vi "系统设置.vi"() -> ()   [LabVIEW 2016]
uses:
  <vilib>/Utility/miscctls.llb/LVPointTypeDef.ctl
  <vilib>/ptbypt/NI_PtbyPt.lvlib
  <vilib>/Utility/config.llb/NI_LVConfig.lvlib
  PLC/PLC.lvlib
  API/CodCr/CodCr.lvlib
panel:
  in  "超标留样启用":bool caption="质控单元禁用"
  in  "周期设置":enum16{"自由设定", "国标协议"}(ring)
  in  "运行间隔":i16=4 min=1 max=24
  out "x = y?":bool
  in  "质控启动日期":string(combo)="关闭"
  in  "跨度核查时间":u16(ring)=6 items=["00H", "01H", "02H", "03H", "04H", "05H", "06H", "07H", "08H", "09H", "10H", "11H", "12H", "13H", "14H", "15H", "16H", "17H", "18H", "19H", "20H", "21H", "22H", "23H"]
  in  "空白核查时间":u16(ring)=2 items=["00H", "01H", "02H", "03H", "04H", "05H", "06H", "07H", "08H", "09H", "10H", "11H", "12H", "13H", "14H", "15H", "16H", "17H", "18H", "19H", "20H", "21H", "22H", "23H"]
  in  "CODCr":bool
  in  "总磷总氮":bool
  in  "氨氮":bool
  in  "CODmn":bool
  in  "多参数":bool
  in  "24H周期设置":bool[](xcontrol)
  in  "输入密码":dbl
  in  "布尔":bool
  in  "副屏设置":bool
  in  "开机启动":bool caption="氨氮禁用"
  in  "CODMn启用":bool caption="CODMn禁用"
  in  "质控单元启用":bool caption="质控单元禁用"
  in  "总磷总氮启用":bool caption="总磷总氮禁用"
  in  "流量计启用":bool caption="流量计禁用"
  in  "氨氮启用":bool caption="氨氮禁用"
  in  "多参数启用":bool caption="多参数禁用"
  in  "CODcr启用":bool caption="CODcr禁用"
  in  "运行模式":enum16{"维护模式", "常规模式", "应急模式", "质控模式"}(ring)
  # "注：周期设置分为自由设定和国标协议两种。\n1：选择自由设定情况下：运行间隔将不可选用并变灰色，周期设置可自由手动勾选\n2：选择国标协议情况下：周期时间将由运行间隔选择的时间决定，下方周期设置被禁用并无法手动勾选。"
  # "自动运行启动参数"
  # "启动周期设置"
  # "质控频次："
  # "空白核查时间："
  # "跨度核查时间："
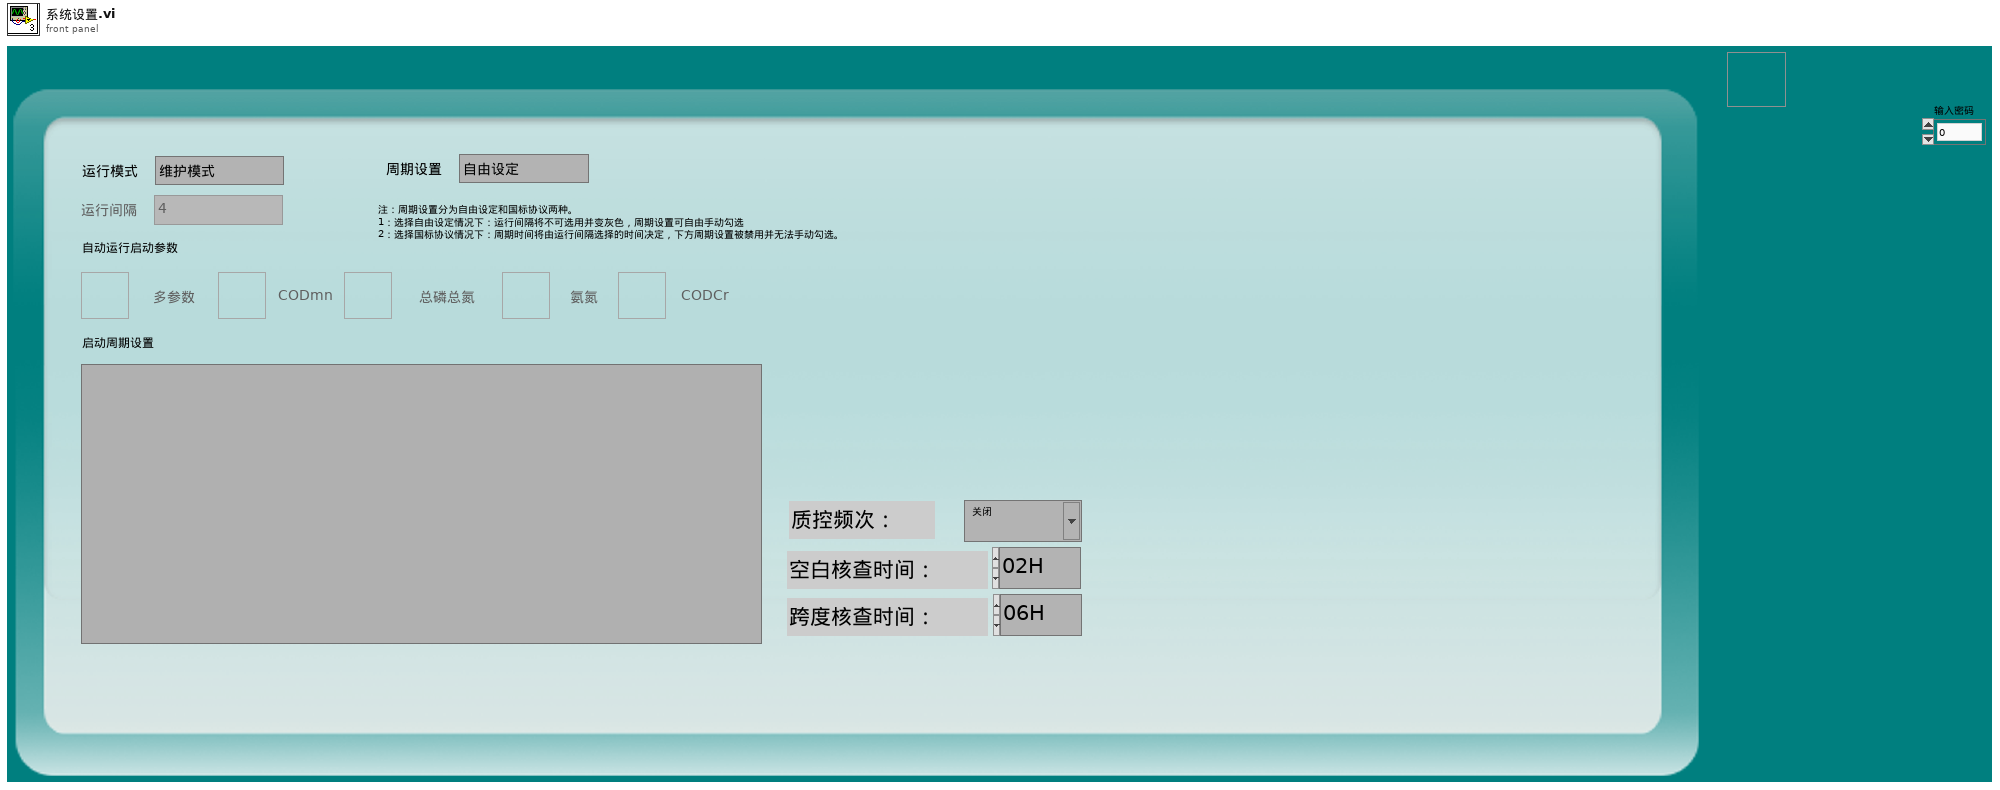
[diagram p1: front panel]
types:
  T1 = typedef "LVPointTypeDef.ctl" = cluster{"Horizontal":i16, "Vertical":i16}
  T2 = typedef "NI_LVConfig.lvlib/Config Data RefNum.ctl" = refnum<k1>
  T3 = enum8{"Enabled", "Disabled", "Disabled and Grayed Out"}
  T4 = enum32{"Invalid", "Standard", "Closed", "Hidden", "Minimized", "Maximized"}
  T5 = enum32{"Bad", "Idle", "Run top level", "Running"}
  T6 = cluster{"运行模式":enum16{"维护模式", "常规模式", "应急模式", "质控模式"}}
  T7 = cluster{"测量模式":enum16{"水样测量", "标样核查", "零点核查", "跨度核查", "加标回收", "平行样", "校零", "校标"}}
  T8 = cluster{"测量模式":enum16{"水样测量", "标样核查", "零点核查", "跨度核查", "空白测试", "加标回收", "平行样", "校零", "校标"}}
  T9 = cluster{"水样测试量程切换模式":enum16{"H", "L", "AUTO"}, "空白核查量程切换模式":enum16{"H", "L", "AUTO"}, "跨度核查量程切换模式":enum16{"H", "L", "AUTO"}}
  T10 = cluster{"站号":u16, "量程切换":enum32{"H", "L", "AUTO"}, "控制命令":enum16{"启动测量", "标样核查", "零点核查", "跨度核查", "空白测试", "平行样测试", "加标回收", "空白校准", "标样校准", "初始化（清洗）", "停止测试", "仪器重启", "校时", "模式设置", "测量间隔设置"}, "模式设置":enum16{"待机", "连续模式", "周期模式", "定点模式", "受控模式", "手动模式"}, "测量间隔":u16}
  T11 = cluster{"CODCr":cluster{"启动测量模式":cluster{"测量模式":enum16{"水样测量", "标样核查", "零点核查", "跨度核查", "加标回收", "平行样", "校零", "校标"}}, "确定按钮":bool}, "参数启用":cluster{"多参数":bool, "CODMn":bool, "总磷总氮":bool, "氨氮":bool, "CODcr":bool}}
  T12 = typedef "LVDateTimeRec.ctl" = cluster{"秒数的小数部分":dbl, "秒":i32, "分":i32, "时":i32, "日":i32, "月":i32, "年":i32, "天数（周）":i32, "天数（年）":i32, "DST":i32}
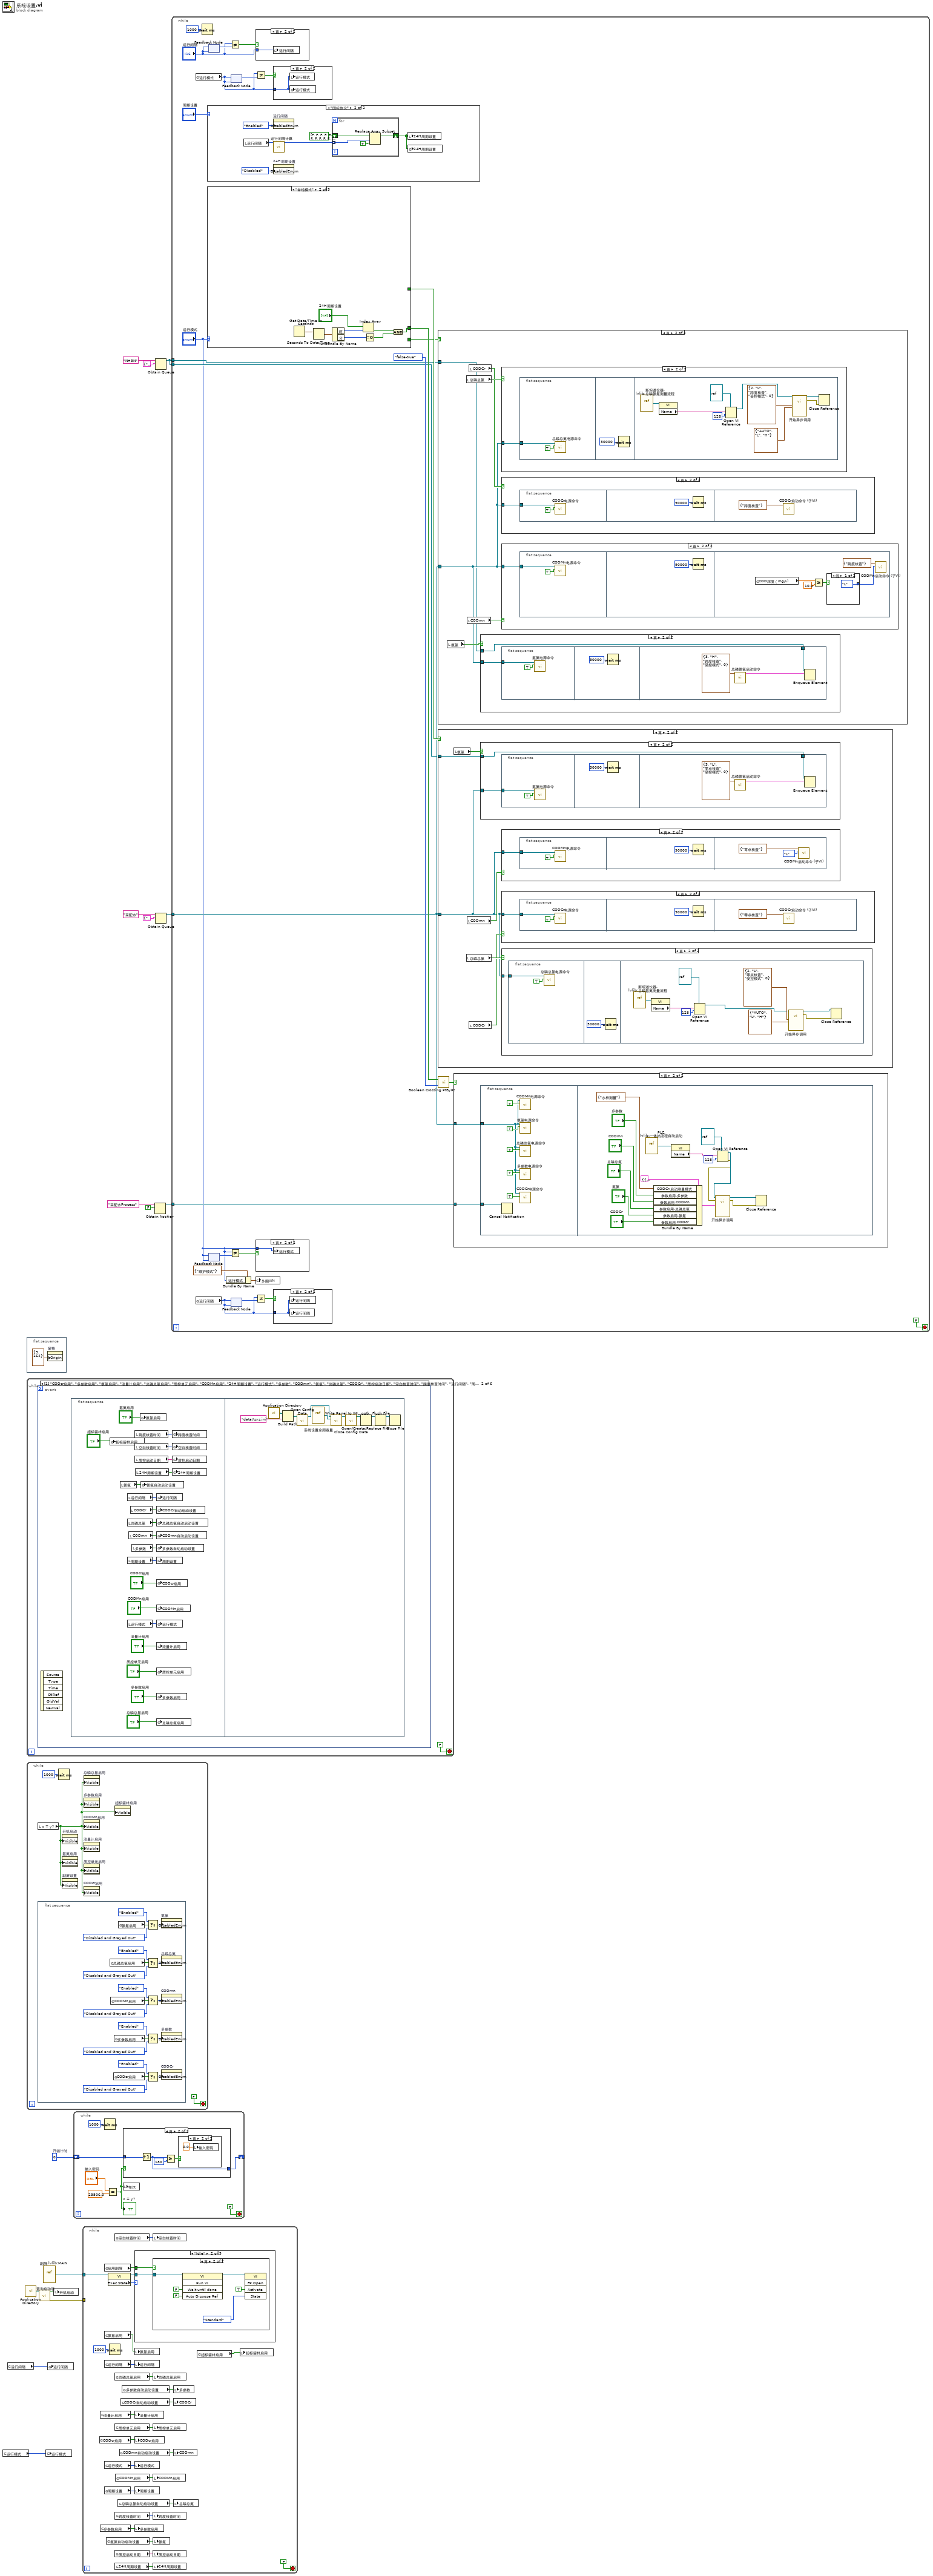
[diagram p0: block diagram]
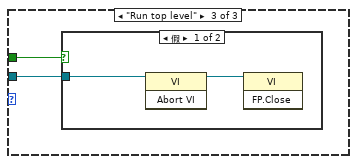
[diagram p6: hidden frame]
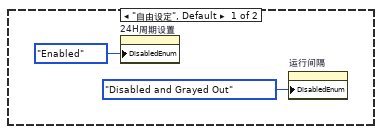
[diagram p8: hidden frame]
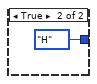
[diagram p16: hidden frame]
diagram:
  w10 = u32 0  # 开锁计时
  n1 = global read "系统设置全局变量.vi" "运行模式"() -> (w2:enum16{"维护模式", "常规模式", "应急模式", "质控模式"})
  n2 = global read "系统设置全局变量.vi" "运行间隔"() -> (w1:i16)
  n3 = call <vilib>:"Application Directory.vi"() -> ("Application Directory"=w13:path)
  n4 = flat-sequence {
    frame #0 {
      n5 = property on="窗格" class="Pane"("Origin"=T1 {"Horizontal"=3, "Vertical"=164} ("原点")) -> ()  [unwired: 2 in, 2 out]
    }
  }
  n6 = while {
    stop <- FALSE stop-if-true
    n7 = event shown="[1] \"CODcr启用\", \"多参数启用\", \"氨氮启用\", \"流量计启用\", \"总磷总氮启用\", \"质控单元启用\", \"CODMn启用\", \"24H周期设置\", \"运行模式\", \"多参数\", \"CODmn\", \"氨氮\", \"总磷总氮\", \"CODCr\", \"质控启动日期\", \"空白核查时间\", \"跨度核查时间\", \"运行间隔\", \"周期设置\", \"超标留样启用\": 值改变" {
      selector: _ -> [_ _ _ _ _ _]
      dyn-events: _ -> [_ _ _ _ _ _]
      timeout: _ -> [_ _ _ _ _ _]
      event Timeout {
        n8 = event-data() -> ()  [unwired: 1 in, 3 out]
      }
      event "CODcr启用", "多参数启用", "氨氮启用", "流量计启用", "总磷总氮启用", "质控单元启用", "CODMn启用", "24H周期设置", "运行模式", "多参数", "CODmn", "氨氮", "总磷总氮", "CODCr", "质控启动日期", "空白核查时间", "跨度核查时间", "运行间隔", "周期设置", "超标留样启用": Value Change {
        n9 = event-data() -> ()  [unwired: 1 in, 6 out]
        n10 = flat-sequence {
          frame #0 {
            n11 = global write "系统设置全局变量.vi" "超标留样启用"("超标留样启用") -> ()
            n12 = local read "氨氮"() -> (w30:bool)
            n13 = local read "运行间隔"() -> (w21:i16)
            n14 = local read "总磷总氮"() -> (w28:bool)
            n15 = local read "周期设置"() -> (w20:enum16{"自由设定", "国标协议"})
            n16 = local read "运行模式"() -> (w31:enum16{"维护模式", "常规模式", "应急模式", "质控模式"})
            n17 = local read "CODmn"() -> (w27:bool)
            n18 = local read "CODCr"() -> (w29:bool)
            n19 = local read "多参数"() -> (w26:bool)
            n20 = local read "跨度核查时间"() -> (w22:u16)
            n21 = local read "空白核查时间"() -> (w23:u16)
            n22 = local read "质控启动日期"() -> (w24:string)
            n23 = local read "24H周期设置"() -> (w25:bool[])
            n24 = global write "系统设置全局变量.vi" "氨氮启用"("氨氮启用") -> ()
            n25 = global write "系统设置全局变量.vi" "氨氮自动启动设置"(w30) -> ()
            n26 = global write "系统设置全局变量.vi" "运行间隔"(w21) -> ()
            n27 = global write "系统设置全局变量.vi" "CODCr自动启动设置"(w29) -> ()
            n28 = global write "系统设置全局变量.vi" "总磷总氮自动启动设置"(w28) -> ()
            n29 = global write "系统设置全局变量.vi" "CODmn自动启动设置"(w27) -> ()
            n30 = global write "系统设置全局变量.vi" "多参数自动启动设置"(w26) -> ()
            n31 = global write "系统设置全局变量.vi" "周期设置"(w20) -> ()
            n32 = global write "系统设置全局变量.vi" "CODcr启用"("CODcr启用") -> ()
            n33 = global write "系统设置全局变量.vi" "CODMn启用"("CODMn启用") -> ()
            n34 = global write "系统设置全局变量.vi" "运行模式"(w31) -> ()
            n35 = global write "系统设置全局变量.vi" "流量计启用"("流量计启用") -> ()
            n36 = global write "系统设置全局变量.vi" "质控单元启用"("质控单元启用") -> ()
            n37 = global write "系统设置全局变量.vi" "多参数启用"("多参数启用") -> ()
            n38 = global write "系统设置全局变量.vi" "总磷总氮启用"("总磷总氮启用") -> ()
            n39 = global write "系统设置全局变量.vi" "跨度核查时间"(w22) -> ()
            n40 = global write "系统设置全局变量.vi" "空白核查时间"(w23) -> ()
            n41 = global write "系统设置全局变量.vi" "质控启动日期"(w24) -> ()
            n42 = global write "系统设置全局变量.vi" "24H周期设置"(w25) -> ()
          }
          frame #1 {
            n43 = call <vilib>:"Application Directory.vi"() -> ("Application Directory"=w52:path)
            n44 = Build Path(base path=w52, name or relative path="data\\sys.ini" ("名称或相对路径")) -> (appended path=w50:path)
            n45 = call <vilib>:"Open Config Data.vi"("configuration file path"=w50) -> ("error out"=w46:errorcluster, "refnum"=w49:T2)  [unwired: 8 in, 1 out]
            n46 = vi-ref "系统设置全局变量.vi"() -> (w48:refnum<vi>)
            n47 = call <userlib>:"Write Panel to INI__ogtk.vi"("error in (no error)"=w46, "VI ref"=w48, "refnum"=w49) -> ("error out"=w45:errorcluster, "refnum out"=w47:T2)  [unwired: 7 in]
            n48 = call <vilib>:"Close Config Data.vi"("error in (no error)"=w45, "refnum"=w47) -> ("error out"=w40:errorcluster, "file path"=w39:path)  [unwired: 8 in]
            n49 = Open/Create/Replace File(file path (use dialog)=w39, error in=w40) -> (refnum out=w43:refnum<file>, error out=w44:errorcluster)  [unwired: 4 in, 1 out]
            n50 = Flush File(refnum=w43, error in=w44) -> (refnum out=w42:refnum<file>, error out=w41:errorcluster)
            n51 = Close File(refnum=w42, error in=w41) -> ()  [unwired: 2 out]
          }
        }
      }
      event "运行间隔": Mouse Down {
        n52 = event-data() -> ("CtlRef"=w56:refnum<vi>)  [unwired: 1 in, 7 out]
        n53 = property class="DigNum (严格)"(reference=w56) -> (reference out=w55:refnum<vi>, "Value"=w54:i16)  [unwired: 1 in, 1 out]
        n54 = call "数字键盘.vi"("OldNumber"=w54) -> ("NewNumber"=w53:sgl)
        n55 = property class="DigNum (严格)"(reference=w55, "Val(Sgnl)"=w53) -> ()  [unwired: 1 in, 2 out]
      }
      event "开机启动": Value Change {
        n56 = event-data() -> ("NewVal"=w58:bool)  [unwired: 1 in, 5 out]
        n57 = call <vilib>:"Application Directory.vi"() -> ("Application Directory"=w57:path)
        n58 = case shown="假" w58 {
          tunnel: w57 -> [w60 w64]
          frame False {
            n59 = call "删除启动项.vi"("启动文件路径"=w60) -> ("删除标记"=w59:bool)  [unwired: 9 in, 1 out]
            n60 = case shown="假" w59 {
              frame False {
                n61 = local write "开机启动"(TRUE ("开机启动")) -> ()
                n62 = One Button Dialog(message="启动项删除失败" ("消息")) -> ()  [unwired: 1 in, 1 out]
              }
              frame True {
              }
            }
          }
          frame True {
            n63 = call "添加启动项.vi"("启动文件路径"=w64) -> ("添加成功标记"=w63:bool)  [unwired: 9 in, 1 out]
            n64 = case shown="假" w63 {
              frame False {
                n65 = local write "开机启动"(FALSE ("开机启动")) -> ()
                n66 = One Button Dialog(message="启动项添加失败" ("消息")) -> ()  [unwired: 1 in, 1 out]
              }
              frame True {
              }
            }
          }
        }
      }
      event "副屏设置": Value Change {
        n67 = event-data() -> ()  [unwired: 1 in, 6 out]
        n68 = call "副屏设置.vi"() -> ()  [unwired: 12 in]
      }
      event "布尔": Value Change {
        n69 = event-data() -> ("OldVal"=w68:bool)  [unwired: 1 in, 5 out]
        n70 = case shown="假" w68 {
          tunnel: [w69 _] -> w67
          frame False {
            n71 = call "数字密码键盘.vi"() -> ("NewNumber"=w69:sgl)  [unwired: 1 in]
          }
          frame True {
          }
        }
        n72 = local write "输入密码"(w67) -> ()
      }
    }
  }
  n73 = while {
    stop <- FALSE stop-if-true
    n74 = local read "x = y?"() -> (w70:bool)
    n75 = flat-sequence {
      frame #0 {
        n76 = global read "系统设置全局变量.vi" "总磷总氮启用"() -> (w79:bool)
        n77 = global read "系统设置全局变量.vi" "CODMn启用"() -> (w77:bool)
        n78 = global read "系统设置全局变量.vi" "CODcr启用"() -> (w78:bool)
        n79 = global read "系统设置全局变量.vi" "多参数启用"() -> (w76:bool)
        n80 = global read "系统设置全局变量.vi" "氨氮启用"() -> (w75:bool)
        n81 = Select(t=T3."Enabled" ("禁用"), s=w75, f=T3."Disabled and Grayed Out" ("禁用")) -> (s? t:f=w80:T3)
        n82 = Select(t=T3."Enabled" ("禁用"), s=w79, f=T3."Disabled and Grayed Out" ("禁用")) -> (s? t:f=w73:T3)
        n83 = Select(t=T3."Enabled" ("禁用"), s=w77, f=T3."Disabled and Grayed Out" ("禁用")) -> (s? t:f=w81:T3)
        n84 = Select(t=T3."Enabled" ("禁用"), s=w76, f=T3."Disabled and Grayed Out" ("禁用")) -> (s? t:f=w74:T3)
        n85 = Select(t=T3."Enabled" ("禁用"), s=w78, f=T3."Disabled and Grayed Out" ("禁用")) -> (s? t:f=w92:T3)
        n86 = property on="氨氮" class="Bool (严格)"("DisabledEnum"=w80) -> ()  [unwired: 2 in, 2 out]
        n87 = property on="总磷总氮" class="Bool (严格)"("DisabledEnum"=w73) -> ()  [unwired: 2 in, 2 out]
        n88 = property on="CODmn" class="Bool (严格)"("DisabledEnum"=w81) -> ()  [unwired: 2 in, 2 out]
        n89 = property on="多参数" class="Bool (严格)"("DisabledEnum"=w74) -> ()  [unwired: 2 in, 2 out]
        n90 = property on="CODCr" class="Bool (严格)"("DisabledEnum"=w92) -> ()  [unwired: 2 in, 2 out]
      }
    }
    n91 = Wait (ms)(milliseconds to wait=u32 1000 ("等待时间（毫秒）")) -> ()  [unwired: 1 out]
    n92 = property on="开机启动" class="Bool (严格)"("Visible"=w70) -> ()  [unwired: 2 in, 2 out]
    n93 = property on="氨氮启用" class="Bool (严格)"("Visible"=w70) -> ()  [unwired: 2 in, 2 out]
    n94 = property on="副屏设置" class="Bool"("Visible"=w70) -> ()  [unwired: 2 in, 2 out]
    n95 = property on="总磷总氮启用" class="Bool (严格)"("Visible"=w70) -> ()  [unwired: 2 in, 2 out]
    n96 = property on="多参数启用" class="Bool (严格)"("Visible"=w70) -> ()  [unwired: 2 in, 2 out]
    n97 = property on="CODMn启用" class="Bool (严格)"("Visible"=w70) -> ()  [unwired: 2 in, 2 out]
    n98 = property on="流量计启用" class="Bool (严格)"("Visible"=w70) -> ()  [unwired: 2 in, 2 out]
    n99 = property on="质控单元启用" class="Bool (严格)"("Visible"=w70) -> ()  [unwired: 2 in, 2 out]
    n100 = property on="CODcr启用" class="Bool (严格)"("Visible"=w70) -> ()  [unwired: 2 in, 2 out]
    n101 = property on="超标留样启用" class="Bool (严格)"("Visible"=w70) -> ()  [unwired: 2 in, 2 out]
  }
  n102 = call "查询启动项.vi"("启动文件路径"=w13) -> ("error out"=w11:errorcluster, "包含启动项"=w12:bool)  [unwired: 9 in]
  n103 = vi-ref "副屏.lvlib:MAIN.vi"() -> (w6:refnum<vi>)
  n104 = global write "系统变量.vi" "运行模式"(w2) -> ()
  n105 = global write "系统变量.vi" "运行间隔"(w1) -> ()
  n106 = local write "开机启动"(w12) -> ()
  n107 = while {
    shift-right: [w94] -> _
    shift-left: w10 -> [w95]
    stop <- FALSE stop-if-true
    n108 = Wait (ms)(milliseconds to wait=u32 1000 ("等待时间（毫秒）")) -> ()  [unwired: 1 out]
    n109 = Equal?(x="输入密码", y=23506.0) -> (x = y?=w93:bool)
    "x = y?" <- w93
    n110 = case shown="真" w93 {
      tunnel: w95 -> [_ w103]
      tunnel: [_ w102] -> w94
      frame False {
      }
      frame True {
        n111 = Increment(x=w103) -> (x+1=w102:u32)
        n112 = Greater Or Equal?(x=w102, y=u32 180) -> (x >= y?=w100:bool)
        n113 = case shown="真" w100 {
          frame False {
          }
          frame True {
            n114 = local write "输入密码"(0.0 ("输入密码")) -> ()
          }
        }
      }
    }
    n115 = local write "布尔"(w93) -> ()
  }
  n116 = while {
    tunnel: w11 -> [_]
    tunnel: w6 -> [w115]
    stop <- FALSE stop-if-true
    n117 = global read "系统设置全局变量.vi" "CODcr启用"() -> (w123:bool)
    n118 = global read "系统设置全局变量.vi" "流量计启用"() -> (w124:bool)
    n119 = global read "系统设置全局变量.vi" "多参数启用"() -> (w122:bool)
    n120 = global read "副屏设置全局变量.vi" "启用副屏"() -> (w113:bool)
    n121 = global read "系统设置全局变量.vi" "氨氮启用"() -> (w128:bool)
    n122 = global read "系统设置全局变量.vi" "运行间隔"() -> (w106:i16)
    n123 = global read "系统设置全局变量.vi" "运行模式"() -> (w105:enum16{"维护模式", "常规模式", "应急模式", "质控模式"})
    n124 = global read "系统设置全局变量.vi" "周期设置"() -> (w108:enum16{"自由设定", "国标协议"})
    n125 = global read "系统设置全局变量.vi" "氨氮自动启动设置"() -> (w120:bool)
    n126 = property class="VI"(reference=w115) -> (reference out=w112:refnum<vi>, "Exec.State"=w114:T5)  [unwired: 1 in, 1 out]
    n127 = Wait (ms)(milliseconds to wait=u32 1000 ("等待时间（毫秒）")) -> ()  [unwired: 1 out]
    n128 = global read "系统设置全局变量.vi" "空白核查时间"() -> (w110:u16)
    n129 = global read "系统设置全局变量.vi" "总磷总氮启用"() -> (w125:bool)
    n130 = global read "系统设置全局变量.vi" "质控单元启用"() -> (w126:bool)
    n131 = global read "系统设置全局变量.vi" "跨度核查时间"() -> (w109:u16)
    n132 = global read "系统设置全局变量.vi" "质控启动日期"() -> (w111:string)
    n133 = global read "系统设置全局变量.vi" "24H周期设置"() -> (w121:bool[])
    n134 = global read "系统设置全局变量.vi" "CODMn启用"() -> (w127:bool)
    n135 = global read "系统设置全局变量.vi" "总磷总氮自动启动设置"() -> (w118:bool)
    n136 = global read "系统设置全局变量.vi" "CODmn自动启动设置"() -> (w117:bool)
    n137 = global read "系统设置全局变量.vi" "CODCr自动启动设置"() -> (w119:bool)
    n138 = global read "系统设置全局变量.vi" "多参数自动启动设置"() -> (w116:bool)
    n139 = case shown="\"Idle\"" w114 {
      tunnel: w113 -> [_ w131 w139]
      tunnel: w112 -> [_ w132 w140]
      frame "Bad", Default {
      }
      frame "Idle" {
        n140 = case shown="真" w131 {
          tunnel: w132 -> [_ w138]
          frame False {
          }
          frame True {
            n141 = invoke class="VI" method="Run VI"(reference=w138, "Wait until done"=FALSE ("结束前等待"), "Auto Dispose Ref"=FALSE ("自动销毁引用")) -> (reference out=w133:refnum<vi>)  [unwired: 2 in, 4 out]
            n142 = invoke class="VI" method="FP.Open"(reference=w133, "Activate"=TRUE ("激活？"), "State"=T4."Standard" ("状态")) -> ()  [unwired: 2 in, 5 out]
          }
        }
      }
      frame "Run top level" {
        n143 = case shown="假" w139 {
          tunnel: w140 -> [w141 _]
          frame False {
            n144 = invoke class="VI" method="Abort VI"(reference=w141) -> (reference out=w142:refnum<vi>)  [unwired: 2 in, 2 out]
            n145 = invoke class="VI" method="FP.Close"(reference=w142) -> ()  [unwired: 2 in, 3 out]
          }
          frame True {
          }
        }
      }
    }
    n146 = local write "氨氮启用"(w128) -> ()
    n147 = local write "运行间隔"(w106) -> ()
    n148 = local write "流量计启用"(w124) -> ()
    n149 = local write "CODcr启用"(w123) -> ()
    n150 = local write "运行模式"(w105) -> ()
    n151 = local write "周期设置"(w108) -> ()
    n152 = local write "多参数启用"(w122) -> ()
    n153 = local write "空白核查时间"(w110) -> ()
    n154 = local write "总磷总氮启用"(w125) -> ()
    n155 = local write "质控单元启用"(w126) -> ()
    n156 = local write "CODMn启用"(w127) -> ()
    n157 = local write "跨度核查时间"(w109) -> ()
    n158 = local write "氨氮"(w120) -> ()
    n159 = local write "质控启动日期"(w111) -> ()
    n160 = local write "24H周期设置"(w121) -> ()
    n161 = local write "多参数"(w116) -> ()
    n162 = local write "CODCr"(w119) -> ()
    n163 = local write "CODmn"(w117) -> ()
    n164 = local write "总磷总氮"(w118) -> ()
    n165 = global read "系统设置全局变量.vi" "超标留样启用"() -> (w107:bool)
    n166 = local write "超标留样启用"(w107) -> ()
  }
  n167 = Obtain Notifier(name (unnamed)="采配水Process" ("名称（未命名）"), notification data type=FALSE) -> (notifier out=w14:refnum<notifier>)  [unwired: 2 in, 2 out]
  n168 = Obtain Queue(name (unnamed)="NH3N" ("名称（未命名）"), element data type=cluster{"命令":string, "data":variant} {"命令"="", "data"=variant}) -> (queue out=w3:refnum<queue>)  [unwired: 3 in, 2 out]
  n169 = Obtain Queue(name (unnamed)="采配水" ("名称（未命名）"), element data type=cluster{"命令":string, "数据":variant} {"命令"="", "数据"=variant}) -> (queue out=w7:refnum<queue>)  [unwired: 3 in, 2 out]
  n170 = while {
    tunnel: w14 -> [w166]
    tunnel: w7 -> [w158]
    tunnel: w3 -> [w157]
    tunnel: w3 -> [w156]
    stop <- FALSE stop-if-true
    n171 = global read "系统变量.vi" "运行模式"() -> (w150:enum16{"维护模式", "常规模式", "应急模式", "质控模式"})
    n172 = global read "系统变量.vi" "运行间隔"() -> (w144:i16)
    n173 = Wait (ms)(milliseconds to wait=u32 1000 ("等待时间（毫秒）")) -> ()  [unwired: 1 out]
    n174 = case shown="\"国标协议\"" "周期设置" {
      frame "自由设定", Default {
        n175 = property on="24H周期设置" class="24H周期设置 (严格)"("DisabledEnum"=T3."Enabled" ("禁用")) -> ()  [unwired: 2 in, 2 out]
        n176 = property on="运行间隔" class="DigNum (严格)"("DisabledEnum"=T3."Disabled and Grayed Out" ("禁用")) -> ()  [unwired: 2 in, 2 out]
      }
      frame "国标协议" {
        n177 = local read "运行间隔"() -> (w176:i16)
        n178 = property on="运行间隔" class="DigNum (严格)"("DisabledEnum"=T3."Enabled" ("禁用")) -> ()  [unwired: 2 in, 2 out]
        n179 = call "运行间隔计算.vi"("运行周期"=w176) -> ("数组"=w175:i32[])  [unwired: 10 in]
        n180 = property on="24H周期设置" class="24H周期设置 (严格)"("DisabledEnum"=T3."Disabled" ("禁用")) -> ()  [unwired: 2 in, 2 out]
        n181 = for {
          tunnel: w175 -> [w179] mode=indexing
          shift-right: [w177] -> w173
          shift-left: bool[] [FALSE, FALSE, FALSE, FALSE, FALSE, FALSE, FALSE, FALSE, FALSE, FALSE, FALSE, FALSE, FALSE, FALSE, FALSE, FALSE, FALSE, FALSE, FALSE, FALSE, FALSE, FALSE, FALSE, FALSE] ("24H周期设置") -> [w180]
          n182 = Replace Array Subset(array=w180, new element=TRUE ("新元素/子数组"), index=w179) -> (w177:bool[])
        }
        n183 = local write "24H周期设置"(w173) -> ()
        n184 = global write "系统设置全局变量.vi" "24H周期设置"(w173) -> ()
      }
    }
    n185 = case shown="\"常规模式\"" "运行模式" {
      tunnel: [_ w294 w301] -> w165
      tunnel: [_ _ w300] -> w159
      tunnel: [_ _ w299] -> w160
      frame "维护模式", Default {
      }
      frame "常规模式" {
        n186 = Get Date/Time In Seconds() -> (seconds since 1Jan1904=w298:timestamp)
        n187 = Seconds To Date/Time(time stamp (now)=w298) -> (date time rec=w297:T12)  [unwired: 1 in]
        n188 = Unbundle By Name(w297) -> ("时"=w292:i32, "分"=w296:i32)
        n189 = Index Array(array="24H周期设置", index=w292) -> (element=w291:bool)
        n190 = Equal To 0?(x=w296) -> (x = 0?=w295:bool)
        n191 = And(x=w291, y=w295) -> (x .and. y?=w294:bool)
      }
      frame "质控模式" {
        n192 = Get Date/Time In Seconds() -> (seconds since 1Jan1904=w309:timestamp)
        n193 = Format Date/Time String(time format string (%c)="%A" ("时间格式字符串(%c)"), seconds (now)=w309) -> (date/time string=w307:string)  [unwired: 1 in]
        n194 = case shown="\"每天\"" "质控启动日期" {
          selector: "质控启动日期" -> [w327 _ _]
          tunnel: [w326 TRUE FALSE] -> w310
          tunnel: w307 -> [w325 _ _]
          frame "星期二", "星期六", "星期日", "星期三", "星期四", "星期五", "星期一" {
            n195 = Equal?(x=w325, y=w327) -> (x = y?=w326:bool)
          }
          frame "每天" {
          }
          frame "关闭", Default {
          }
        }
        n196 = local read "24H周期设置"() -> (w304:bool[])
        n197 = Seconds To Date/Time(time stamp (now)=w309) -> (date time rec=w324:T12)  [unwired: 1 in]
        n198 = Unbundle By Name(w324) -> ("时"=w302:i32, "分"=w323:i32, "时"=w321:i32, "分"=w319:i32, "时"=w315:i32, "分"=w314:i32, "秒"=w306:i32)
        n199 = Equal?(x=w321, y="空白核查时间") -> (x = y?=w318:bool)
        n200 = Equal?(x=w315, y="跨度核查时间") -> (x = y?=w313:bool)
        n201 = Index Array(array=w304, index=w302) -> (element=w303:bool)
        n202 = Equal To 0?(x=w323) -> (x = 0?=w322:bool)
        n203 = Equal To 0?(x=w319) -> (x = 0?=w317:bool)
        n204 = Equal To 0?(x=w314) -> (x = 0?=w312:bool)
        n205 = Equal To 0?(x=w306) -> (x = 0?=w305:bool)
        n206 = And(x=w303, y=w322) -> (x .and. y?=w301:bool)
        n207 = Compound Arithmetic op=AND ("复合运算")(w317, w318, w310, w305) -> (w299:bool)
        n208 = Compound Arithmetic op=AND ("复合运算")(w313, w312, w310, w305) -> (w300:bool)
      }
    }
    n209 = feedback #1("运行间隔") -> (w149:i16)
    n210 = feedback-in #1("运行间隔") -> ()
    n211 = feedback-in #2("运行模式") -> ()
    n212 = feedback #2("运行模式") -> (w155:enum16{"维护模式", "常规模式", "应急模式", "质控模式"})
    n213 = Bundle By Name(cluster=T6 {"运行模式"=enum."维护模式"} ("外围API"), "运行模式"="运行模式") -> (w161:T6)
    n214 = Not Equal?(x="运行间隔", y=w149) -> (x != y?=w148:bool)
    n215 = Not Equal?(x="运行模式", y=w155) -> (x != y?=w154:bool)
    n216 = feedback #3(w150) -> (w152:enum16{"维护模式", "常规模式", "应急模式", "质控模式"})
    n217 = feedback-in #3(w150) -> ()
    n218 = feedback #4(w144) -> (w146:i16)
    n219 = feedback-in #4(w144) -> ()
    n220 = case shown="真" w148 {
      tunnel: "运行间隔" -> [_ w182]
      frame False {
      }
      frame True {
        n221 = global write "系统变量.vi" "运行间隔"(w182) -> ()
      }
    }
    n222 = Not Equal?(x=w150, y=w152) -> (x != y?=w151:bool)
    n223 = case shown="真" w154 {
      tunnel: "运行模式" -> [_ w184]
      frame False {
      }
      frame True {
        n224 = global write "系统变量.vi" "运行模式"(w184) -> ()
      }
    }
    n225 = global write "VAR总磷氨氮全局变量.vi" "外围API"(w161) -> ()
    n226 = Not Equal?(x=w144, y=w146) -> (x != y?=w145:bool)
    n227 = case shown="真" w151 {
      tunnel: w150 -> [_ w183]
      frame False {
      }
      frame True {
        n228 = local write "运行模式"(w183) -> ()
        n229 = global write "系统设置全局变量.vi" "运行模式"(w183) -> ()
      }
    }
    n230 = case shown="真" w145 {
      tunnel: w144 -> [_ w181]
      frame False {
      }
      frame True {
        n231 = global write "系统设置全局变量.vi" "运行间隔"(w181) -> ()
        n232 = local write "运行间隔"(w181) -> ()
      }
    }
    n233 = case shown="真" w159 {
      tunnel: w158 -> [_ w186]
      tunnel: w156 -> [_ w185]
      frame False {
      }
      frame True {
        n234 = local read "氨氮"() -> (w190:bool)
        n235 = local read "总磷总氮"() -> (w189:bool)
        n236 = local read "CODmn"() -> (w188:bool)
        n237 = local read "CODCr"() -> (w187:bool)
        n238 = case shown="真" w190 {
          tunnel: w186 -> [_ w221]
          tunnel: w185 -> [_ w220]
          frame False {
          }
          frame True {
            n239 = flat-sequence {
              tunnel: w221 -> [w222]
              tunnel: w220 -> [w225]
              frame #0 {
                n240 = call "氨氮电源命令.vi"("通电/断电"=TRUE, "队列"=w222) -> ()  [unwired: 9 in, 1 out]
              }
              frame #1 {
                n241 = Wait (ms)(milliseconds to wait=u32 30000 ("等待时间（毫秒）")) -> ()  [unwired: 1 out]
              }
              frame #2 {
                n242 = call "总磷氨氮启动命令.vi"("参数"=T10 {"站号"=3, "量程切换"=enum."H", "控制命令"=enum."跨度核查", "模式设置"=enum."受控模式", "测量间隔"=0}) -> ("启动命令"=w227:cluster{"命令":string, "data":variant})  [unwired: 10 in]
                n243 = Enqueue Element(queue=w225, element=w227) -> ()  [unwired: 2 in, 3 out]
              }
            }
          }
        }
        n244 = case shown="真" w189 {
          tunnel: w186 -> [_ w207]
          frame False {
          }
          frame True {
            n245 = flat-sequence {
              tunnel: w207 -> [w209]
              frame #0 {
                n246 = call "总磷总氮电源命令.vi"("通电/断电"=TRUE, "队列"=w209) -> ()  [unwired: 9 in, 1 out]
              }
              frame #1 {
                n247 = Wait (ms)(milliseconds to wait=u32 30000 ("等待时间（毫秒）")) -> ()  [unwired: 1 out]
              }
              frame #2 {
                n248 = vi-ref "斯坦道仪器.lvlib:总磷氨氮测量流程.vi"() -> (w216:refnum<vi>)
                n249 = property class="VI"(reference=w216) -> ("Name"=w217:string)  [unwired: 1 in, 2 out]
                n250 = Open VI Reference(type specifier VI Refnum (for type only)=refnum<vi> refnum ("类型说明符VI引用句柄（仅用于类型）"), vi path=w217, options=128 ("选项")) -> (vi reference=w215:refnum<vi>)  [unwired: 3 in, 1 out]
                n251 = call-by-ref "开始异步调用"(reference=w215, "量程模式"=T9 {"水样测试量程切换模式"=enum."AUTO", "空白核查量程切换模式"=enum."L", "跨度核查量程切换模式"=enum."H"}, "参数"=T10 {"站号"=2, "量程切换"=enum."L", "控制命令"=enum."跨度核查", "模式设置"=enum."受控模式", "测量间隔"=0}) -> (reference out=w212:refnum<vi>, error out=w211:errorcluster)  [unwired: 11 in]
                n252 = Close Reference(reference=w212, error in (no error)=w211) -> ()  [unwired: 1 out]
              }
            }
          }
        }
        n253 = case shown="真" w187 {
          tunnel: w186 -> [_ w191]
          frame False {
          }
          frame True {
            n254 = flat-sequence {
              tunnel: w191 -> [w192]
              frame #0 {
                n255 = call "CODCr电源命令.vi"("通电/断电"=TRUE, "队列"=w192) -> ()  [unwired: 9 in, 1 out]
              }
              frame #1 {
                n256 = Wait (ms)(milliseconds to wait=u32 90000 ("等待时间（毫秒）")) -> ()  [unwired: 1 out]
              }
              frame #2 {
                n257 = call "CODCr启动命令 (子VI).vi"("启动测量模式"=T7 {"测量模式"=enum."跨度核查"}) -> ()  [unwired: 11 in]
              }
            }
          }
        }
        n258 = case shown="真" w188 {
          tunnel: w186 -> [_ w196]
          frame False {
          }
          frame True {
            n259 = flat-sequence {
              tunnel: w196 -> [w197]
              frame #0 {
                n260 = call "CODMn电源命令.vi"("通电/断电"=TRUE, "队列"=w197) -> ()  [unwired: 9 in, 1 out]
              }
              frame #1 {
                n261 = Wait (ms)(milliseconds to wait=u32 90000 ("等待时间（毫秒）")) -> ()  [unwired: 1 out]
              }
              frame #2 {
                n262 = global read "COD浓度全局变量.vi" "COD浓度（mg/L)"() -> (w201:dbl)
                n263 = Greater Or Equal?(x=w201, y=10.0) -> (x >= y?=w203:bool)
                n264 = case shown="假" w203 {
                  tunnel: [enum32{"H", "L", "AUTO"}."L" ("CODMn量程切换") enum32{"H", "L", "AUTO"}."H" ("CODMn量程切换")] -> w200
                  frame False {
                  }
                  frame True {
                  }
                }
                n265 = call "CODMn启动命令 (子VI).vi"("CODMn量程切换"=w200, "启动测量模式"=T8 {"测量模式"=enum."跨度核查"}) -> ()  [unwired: 10 in]
              }
            }
          }
        }
      }
    }
    n266 = case shown="真" w160 {
      tunnel: w158 -> [_ w229]
      tunnel: w157 -> [_ w228]
      frame False {
      }
      frame True {
        n267 = local read "氨氮"() -> (w233:bool)
        n268 = local read "总磷总氮"() -> (w232:bool)
        n269 = local read "CODmn"() -> (w231:bool)
        n270 = local read "CODCr"() -> (w230:bool)
        n271 = case shown="真" w233 {
          tunnel: w229 -> [_ w259]
          tunnel: w228 -> [_ w258]
          frame False {
          }
          frame True {
            n272 = flat-sequence {
              tunnel: w259 -> [w260]
              tunnel: w258 -> [w263]
              frame #0 {
                n273 = call "氨氮电源命令.vi"("通电/断电"=TRUE, "队列"=w260) -> ()  [unwired: 9 in, 1 out]
              }
              frame #1 {
                n274 = Wait (ms)(milliseconds to wait=u32 30000 ("等待时间（毫秒）")) -> ()  [unwired: 1 out]
              }
              frame #2 {
                n275 = call "总磷氨氮启动命令.vi"("参数"=T10 {"站号"=3, "量程切换"=enum."L", "控制命令"=enum."零点核查", "模式设置"=enum."受控模式", "测量间隔"=0}) -> ("启动命令"=w264:cluster{"命令":string, "data":variant})  [unwired: 10 in]
                n276 = Enqueue Element(queue=w263, element=w264) -> ()  [unwired: 2 in, 3 out]
              }
            }
          }
        }
        n277 = case shown="真" w231 {
          tunnel: w229 -> [_ w239]
          frame False {
          }
          frame True {
            n278 = flat-sequence {
              tunnel: w239 -> [w240]
              frame #0 {
                n279 = call "CODMn电源命令.vi"("通电/断电"=TRUE, "队列"=w240) -> ()  [unwired: 9 in, 1 out]
              }
              frame #1 {
                n280 = Wait (ms)(milliseconds to wait=u32 90000 ("等待时间（毫秒）")) -> ()  [unwired: 1 out]
              }
              frame #2 {
                n281 = call "CODMn启动命令 (子VI).vi"("CODMn量程切换"=enum32{"H", "L", "AUTO"}."L", "启动测量模式"=T8 {"测量模式"=enum."零点核查"}) -> ()  [unwired: 10 in]
              }
            }
          }
        }
        n282 = case shown="真" w230 {
          tunnel: w229 -> [_ w234]
          frame False {
          }
          frame True {
            n283 = flat-sequence {
              tunnel: w234 -> [w235]
              frame #0 {
                n284 = call "CODCr电源命令.vi"("通电/断电"=TRUE, "队列"=w235) -> ()  [unwired: 9 in, 1 out]
              }
              frame #1 {
                n285 = Wait (ms)(milliseconds to wait=u32 90000 ("等待时间（毫秒）")) -> ()  [unwired: 1 out]
              }
              frame #2 {
                n286 = call "CODCr启动命令 (子VI).vi"("启动测量模式"=T7 {"测量模式"=enum."零点核查"}) -> ()  [unwired: 11 in]
              }
            }
          }
        }
        n287 = case shown="真" w232 {
          tunnel: w229 -> [_ w245]
          frame False {
          }
          frame True {
            n288 = flat-sequence {
              tunnel: w245 -> [w247]
              frame #0 {
                n289 = call "总磷总氮电源命令.vi"("通电/断电"=TRUE, "队列"=w247) -> ()  [unwired: 9 in, 1 out]
              }
              frame #1 {
                n290 = Wait (ms)(milliseconds to wait=u32 30000 ("等待时间（毫秒）")) -> ()  [unwired: 1 out]
              }
              frame #2 {
                n291 = vi-ref "斯坦道仪器.lvlib:总磷氨氮测量流程.vi"() -> (w253:refnum<vi>)
                n292 = property class="VI"(reference=w253) -> ("Name"=w254:string)  [unwired: 1 in, 2 out]
                n293 = Open VI Reference(type specifier VI Refnum (for type only)=refnum<vi> refnum ("类型说明符VI引用句柄（仅用于类型）"), vi path=w254, options=128 ("选项")) -> (vi reference=w251:refnum<vi>)  [unwired: 3 in, 1 out]
                n294 = call-by-ref "开始异步调用"(reference=w251, "量程模式"=T9 {"水样测试量程切换模式"=enum."AUTO", "空白核查量程切换模式"=enum."L", "跨度核查量程切换模式"=enum."H"}, "参数"=T10 {"站号"=2, "量程切换"=enum."L", "控制命令"=enum."零点核查", "模式设置"=enum."受控模式", "测量间隔"=0}) -> (reference out=w250:refnum<vi>, error out=w249:errorcluster)  [unwired: 11 in]
                n295 = Close Reference(reference=w250, error in (no error)=w249) -> ()  [unwired: 1 out]
              }
            }
          }
        }
      }
    }
    n296 = call <vilib>:"Boolean Crossing PtByPt.vi"("direction"=enum16{"either", "false-true", "true-false"}."false-true", "input"=w165) -> ("crossing"=w163:bool)  [unwired: 1 in]
    n297 = case shown="真" w163 {
      tunnel: w166 -> [_ w267]
      tunnel: w158 -> [_ w266]
      frame False {
      }
      frame True {
        n298 = flat-sequence {
          tunnel: w267 -> [w274]
          tunnel: w266 -> [w268]
          frame #0 {
            n299 = Cancel Notification(0:w274) -> ()  [unwired: 1 in, 3 out]
            n300 = call "CODMn电源命令.vi"("通电/断电"=TRUE, "队列"=w268) -> ()  [unwired: 9 in, 1 out]
            n301 = call "氨氮电源命令.vi"("通电/断电"=TRUE, "队列"=w268) -> ()  [unwired: 9 in, 1 out]
            n302 = call "总磷总氮电源命令.vi"("通电/断电"=TRUE, "队列"=w268) -> ()  [unwired: 9 in, 1 out]
            n303 = call "多参数电源命令.vi"("通电/断电"=TRUE, "队列"=w268) -> ()  [unwired: 9 in, 1 out]
            n304 = call "CODCr电源命令.vi"("通电/断电"=TRUE, "队列"=w268) -> ()  [unwired: 9 in, 1 out]
          }
          frame #1 {
            n305 = vi-ref "PLC.lvlib:一体站流程自动启动.vi"() -> (w280:refnum<vi>)
            n306 = Bundle By Name(cluster=T11 {"CODCr"={"启动测量模式"={"测量模式"=enum."水样测量"}, "确定按钮"=FALSE}, "参数启用"={"多参数"=FALSE, "CODMn"=FALSE, "总磷总氮"=FALSE, "氨氮"=FALSE, "CODcr"=FALSE}} ("参数"), "CODCr.启动测量模式"=T7 {"测量模式"=enum."水样测量"}, "参数启用.多参数"="多参数", "参数启用.CODMn"="CODmn", "参数启用.总磷总氮"="总磷总氮", "参数启用.氨氮"="氨氮", "参数启用.CODcr"="CODCr") -> (w284:T11)
            n307 = property class="VI"(reference=w280) -> ("Name"=w281:string)  [unwired: 1 in, 2 out]
            n308 = Open VI Reference(type specifier VI Refnum (for type only)=refnum<vi> refnum ("类型说明符VI引用句柄（仅用于类型）"), vi path=w281, options=128 ("选项")) -> (vi reference=w278:refnum<vi>, error out=w277:errorcluster)  [unwired: 3 in]
            n309 = call-by-ref "开始异步调用"(reference=w278, error in=w277, "参数"=w284) -> (reference out=w276:refnum<vi>, error out=w275:errorcluster)  [unwired: 11 in]
            n310 = Close Reference(reference=w276, error in (no error)=w275) -> ()  [unwired: 1 out]
          }
        }
      }
    }
  }
